vi "SENS_SWE_TRIG_POIN_ON_OFF.vi"(0 "VISA IN":refnum<visa-resource-name>, 1 "One data point? ON/OFF":bool, 5 "error in":errorcluster, 7 "Channel":i32) -> (14 "VISA Out":refnum<visa-resource-name>, 19 "error out":errorcluster)   [LabVIEW 2018, in "PNA-X.lvlib"]
doc: "SENSe<cnum>:SWEep:TRIGger:POINt <ON | OFF> \n(Read-Write) Specifies whether the specified channel will measure one point for each trigger or all of the \nmeasurements in the channel. Setting any channel to POINt mode will automatically set the TRIGger:SCOPe = \nCURRent.\nParameters \n<cnum> Any existing channel number. If unspecified, value is set to 1 \n<ON | OFF> ON (or 1) - Channel measures one data point per trigger. \nOFF (or 0) - All measurements in the channel made per trigger. \nExamples SENS:SWE:TRIG:POIN ON \nsense2:sweep:trigger:point off \nQuery Syntax SENSe<cnum>:SWEep:TRIGger:POINt? \nReturn Type Boolean (1 = Point, 0 = Measurement) \nDefault 0 - Measurement"
uses:
  PNA-X.lvlib
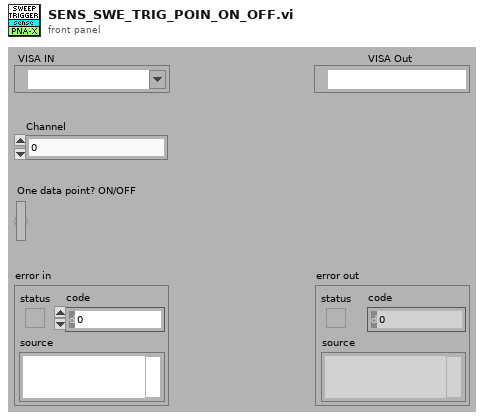
[diagram p1: front panel]
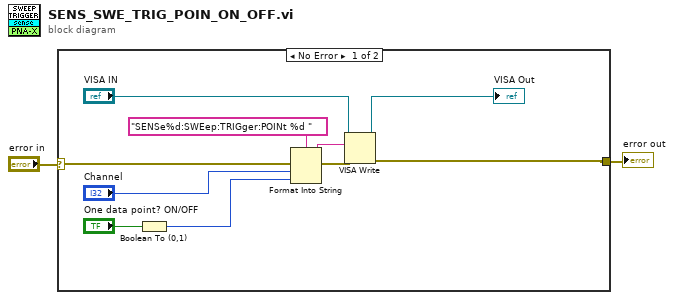
[diagram p0: block diagram]
diagram:
  n1 = case shown="No Error" "error in" {
    selector: "error in" -> [w12 w13]
    tunnel: [w7 w13] -> w1
    frame No Error {
      n2 = Boolean To (0,1)(Boolean="One data point? ON/OFF") -> (0, 1=w3:i16)
      n3 = Format Into String(format string="SENSe%d:SWEep:TRIGger:POINt %d " ("Cmdline"), error in=w12, "Channel", w3) -> (resulting string=w10:string, error out=w11:errorcluster)  [unwired: 1 in]
      n4 = VISA Write(VISA resource name="VISA IN", write buffer=w10, error in (no error)=w11) -> (VISA resource name out=→"VISA Out":refnum<visa-resource-name>, error out=w7:errorcluster)  [unwired: 1 out]
    }
    frame Error {
    }
  }
  "error out" <- w1
